vi "Status.vi"() -> ()   [LabVIEW 2019]
panel:
  in  "Skip Next Dose":bool
  in  "Retain Next Dose":bool
  in  "BoosterDosageMessage":string
  in  "Booster2":timestamp=timestamp(3660681600 s since 1904-01-01) format="%<%d/%m/%y %I:%M %p>T"
  in  "Booster1":timestamp=timestamp(3660681600 s since 1904-01-01) format="%<%d/%m/%y %I:%M %p>T"
  in  "Dose10":timestamp=timestamp(3660681600 s since 1904-01-01) format="%<%d/%m/%y %I:%M %p>T"
  in  "Dose9":timestamp=timestamp(3660681600 s since 1904-01-01) format="%<%d/%m/%y %I:%M %p>T"
  in  "Dose8":timestamp=timestamp(3660681600 s since 1904-01-01) format="%<%d/%m/%y %I:%M %p>T"
  in  "Dose7":timestamp=timestamp(3660681600 s since 1904-01-01) format="%<%d/%m/%y %I:%M %p>T"
  in  "Dose6":timestamp=timestamp(3660681600 s since 1904-01-01) format="%<%d/%m/%y %I:%M %p>T"
  in  "Dose5":timestamp=timestamp(3660681600 s since 1904-01-01) format="%<%d/%m/%y %I:%M %p>T"
  in  "Dose4":timestamp=timestamp(3660681600 s since 1904-01-01) format="%<%d/%m/%y %I:%M %p>T"
  in  "Dose3":timestamp=timestamp(3660681600 s since 1904-01-01) format="%<%d/%m/%y %I:%M %p>T"
  in  "Dose2":timestamp=timestamp(3660681600 s since 1904-01-01) format="%<%d/%m/%y %I:%M %p>T"
  in  "Dose1":timestamp=timestamp(3660681600 s since 1904-01-01) format="%<%d/%m/%y %I:%M %p>T"
  # "Randoly Generated Booster Doses"
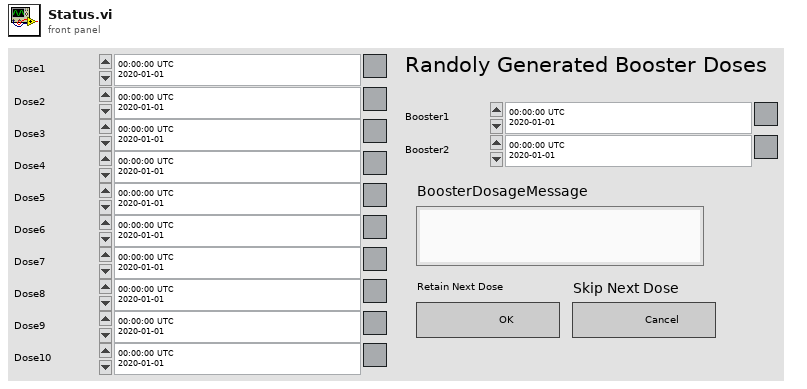
[diagram p1: front panel]
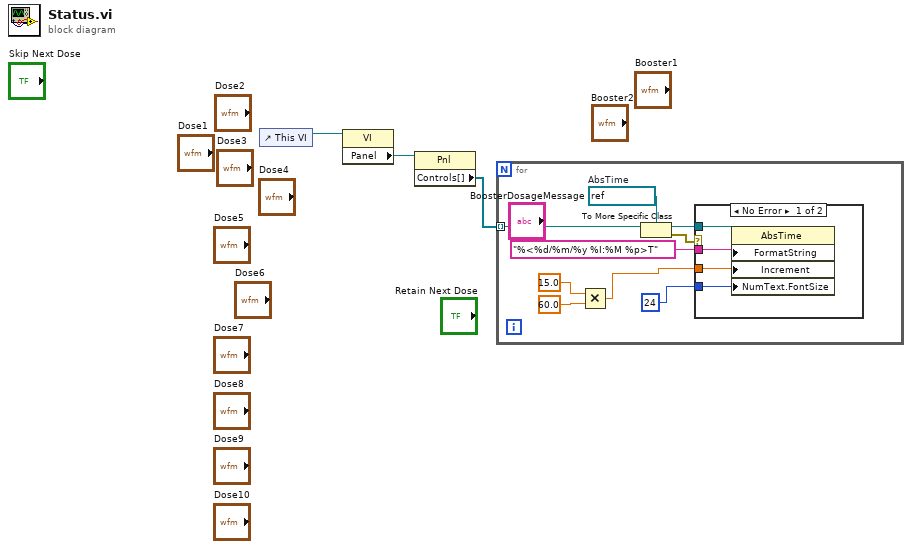
[diagram p0: block diagram]
diagram:
  n1 = control-ref of="This VI"() -> (w3:refnum<vi>)
  n2 = property class="VI"(reference=w3) -> ("Panel"=w2:refnum<vi>)  [unwired: 1 in, 2 out]
  n3 = property class="Pnl"(reference=w2) -> ("Controls[]"=w1:refnum<vi>[])  [unwired: 1 in, 2 out]
  n4 = for {
    tunnel: w1 -> [w12] mode=indexing
    w11 = refnum<vi> refnum  # AbsTime
    n5 = Multiply(x=15.0, y=60.0) -> (x*y=w4:dbl)
    n6 = To More Specific Class(target class=w11, reference=w12) -> (specific class reference=w10:refnum<vi>, error out=w8:errorcluster)  [unwired: 1 in]
    n7 = case shown="No Error" w8 {
      tunnel: w10 -> [w16 _]
      tunnel: "%<%d/%m/%y %I:%M %p>T" ("Format String") -> [w15 _]
      tunnel: w4 -> [w14 _]
      tunnel: u32 24 ("Numeric Text.Font:Size") -> [w13 _]
      frame No Error {
        n8 = property class="AbsTime"(reference=w16, "FormatString"=w15, "Increment"=w14, "NumText.FontSize"=w13) -> ()  [unwired: 1 in, 2 out]
      }
      frame Error {
      }
    }
  }
